vi "nxt main.vi"() -> ()   [LabVIEW 2012, in "Tugboat.lvrbt"]
uses:
  Tugboat.lvrbt
  tugProperties_t.ctl
  sensorData_t.ctl
  irData_t.ctl
  motorData_t.ctl
  motorCommands_t.ctl
  <vilib>/NXT/Block Support/NXT_TimerIndex.ctl
  behaviorWeights_t.ctl
panel:
  in  "_sendToPC":string
  in  "_fromPC":u8[](array[numeric])=[0, 0, 0, 0, 0, 0, 0, 0, 0, 0, 0]
  out "Sense/Act":bool=TRUE
  in  "_motorCommands":T1={"_rudderCommand"=7, "_propCommand"=7, "_irServoCommand"=7}
  in  "_motorData":T2={"_rudderCommand"=1450, "_propCommand"=1500, "_irServoCommand"=1550}
  in  "_sensorData":T3={"_irData"={"_irDistance"=0, "_irHeading"=0, "_irTimestamp"=0}, "_batteryVoltage"=0, "_NXTButtonStates"=[FALSE, FALSE, FALSE]}
  in  "Tugboat Properties":T5={"_name"="Enterprise", "_pitch"=440, "_rudderCenter"=1450, "_propCenter"=1500, "_irServoCenter"=1550, "_rudderMin"=930, "_rudderMax"=2000, "_propMin"=1000, "_propMax"=2000, "_irServoMin"=800, "_irServoMax"=2200}
  in  "SOFT E-STOP":bool
  in  "HARD E-STOP":bool
  # "L\nE\nF\nT"
  # "C\nE\nN\nT\nE\nR"
  # "R\nI\nG\nH\nT"
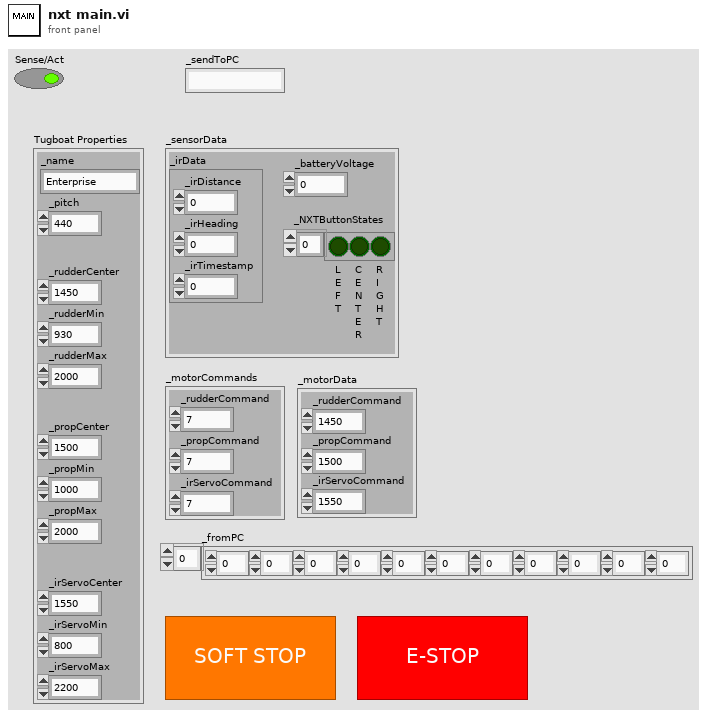
[diagram p1: front panel]
types:
  T1 = typedef "motorCommands_t.ctl" = cluster{"_rudderCommand":i8, "_propCommand":i8, "_irServoCommand":i8}
  T2 = typedef "motorData_t.ctl" = cluster{"_rudderCommand":u16, "_propCommand":u16, "_irServoCommand":u16}
  T3 = typedef "sensorData_t.ctl" = cluster{"_irData":T4, "_batteryVoltage":i32, "_NXTButtonStates":bool[]}
  T4 = typedef "irData_t.ctl" = cluster{"_irDistance":i32, "_irHeading":i32, "_irTimestamp":u32}
  T5 = typedef "tugProperties_t.ctl" = cluster{"_name":string, "_pitch":i32, "_rudderCenter":u16, "_propCenter":u16, "_irServoCenter":u16, "_rudderMin":u16, "_rudderMax":u16, "_propMin":u16, "_propMax":u16, "_irServoMin":u16, "_irServoMax":u16}
  T6 = typedef "behaviorWeights_t.ctl" = i8[]
  T7 = typedef "NXT_TimerIndex.ctl" = u8
  T8 = typedef "LVHSConnector.ctl" = cluster{"Hardware":string, "Flattened String":string}
  T9 = typedef "behaviorOutput_t.ctl" = cluster{"Goodness":i8[], "Velocity":i8[], "Weight":i8}
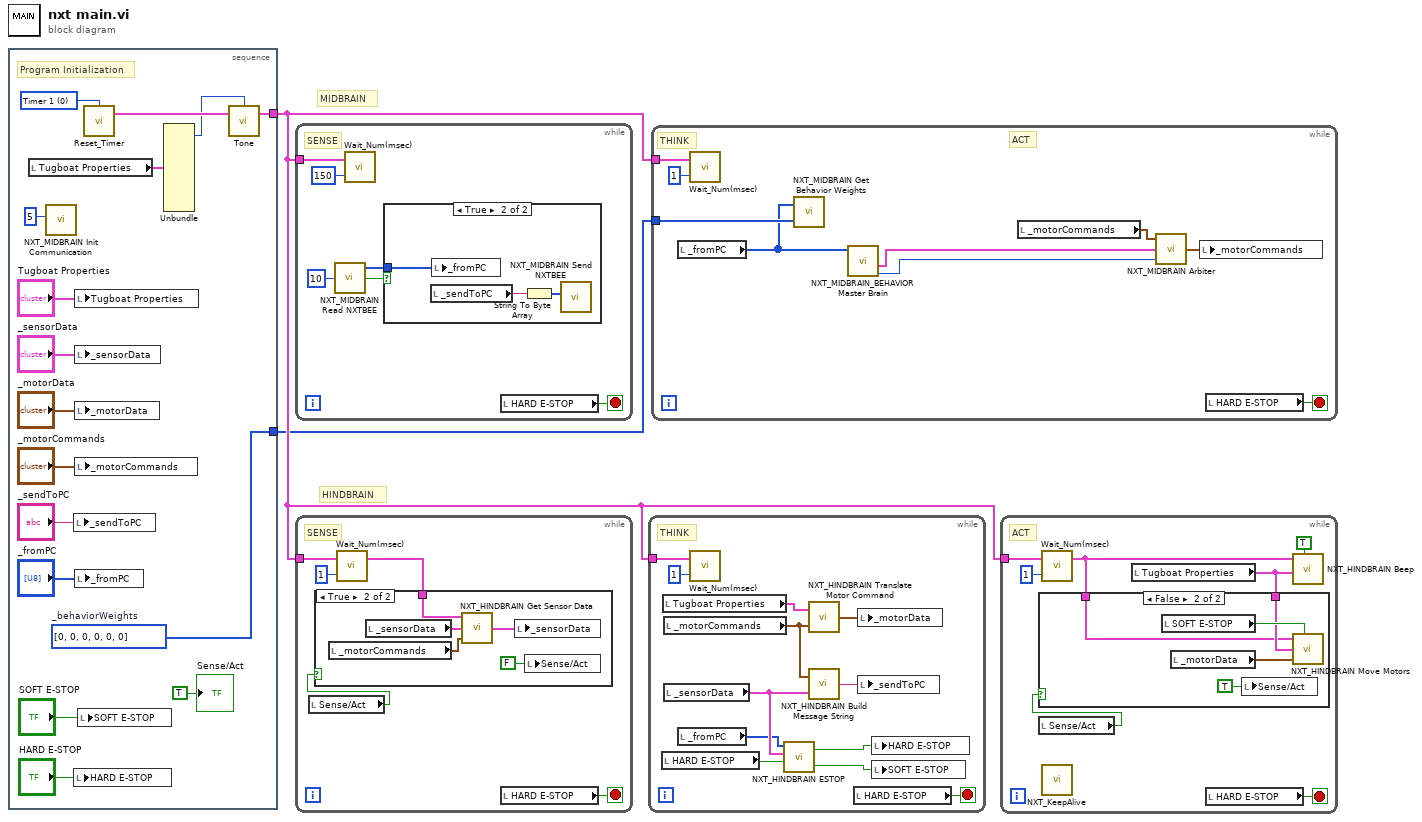
[diagram p0: block diagram]
diagram:
  # "HINDBRAIN"
  # "MIDBRAIN"
  n1 = stacked-sequence {
    tunnel: [w12] -> w2
    tunnel: [w6] -> w1
    frame #0 {
      w6 = T6 [0, 0, 0, 0, 0, 0]  # _behaviorWeights
      w14 = T7 0 items=["Timer 1", "Timer 2", "Timer 3"] ("Timer (Timer 1)")
      # "Program Initialization"
      n2 = local read "Tugboat Properties"() -> (w17:T5)
      n3 = call "NXT_MIDBRAIN Init Communication.vi"("Speed"=u8 5) -> ()  [unwired: 6 in, 1 out]
      n4 = local write "_sendToPC"("_sendToPC") -> ()
      n5 = local write "HARD E-STOP"("HARD E-STOP") -> ()
      n6 = local write "Tugboat Properties"("Tugboat Properties") -> ()
      n7 = local write "_sensorData"("_sensorData") -> ()
      n8 = local write "_motorData"("_motorData") -> ()
      n9 = local write "_motorCommands"("_motorCommands") -> ()
      n10 = local write "_fromPC"("_fromPC") -> ()
      n11 = local write "SOFT E-STOP"("SOFT E-STOP") -> ()
      n12 = call <vilib>:"Reset_Timer.vi"("Timer (Timer 1)"=w14) -> ("NXT"=w9:T8)  [unwired: 3 in]
      n13 = Unbundle(w17) -> ("_pitch"=w7:i32)  [unwired: 10 out]
      n14 = call <vilib>:"Tone.vi"("NXT"=w9, "Tone (440 Hz)"=w7) -> ("NXT"=w12:T8)  [unwired: 2 in]
      "Sense/Act" <- TRUE ("Sense/Act")
    }
  }
  n15 = while {
    tunnel: w2 -> [w23]
    stop <- w22 stop-if-true
    # "SENSE"
    n16 = call "NXT_MIDBRAIN Read NXTBEE.vi"("#bytes"=u8 10) -> ("Valid String?"=w19:bool, "Data Out"=w21:u8[])  [unwired: 2 in, 1 out]
    n17 = call <vilib>:"Wait_Num(msec).vi"("Time (100 msec)"=u32 150, "NXT"=w23) -> ()  [unwired: 2 in, 1 out]
    n18 = case shown="True" w19 {
      tunnel: w21 -> [_ w25]
      frame False {
      }
      frame True {
        n19 = local read "_sendToPC"() -> (w26:string)
        n20 = local write "_fromPC"(w25) -> ()
        n21 = String To Byte Array(string=w26) -> (unsigned byte array=w27:u8[])
        n22 = call "NXT_MIDBRAIN Send NXTBEE.vi"("Data"=w27) -> ()  [unwired: 8 in, 1 out]
      }
    }
    n23 = local read "HARD E-STOP"() -> (w22:bool)
  }
  n24 = while {
    tunnel: w2 -> [w29]
    stop <- w31 stop-if-true
    # "SENSE"
    n25 = local read "Sense/Act"() -> (w28:bool)
    n26 = call <vilib>:"Wait_Num(msec).vi"("Time (100 msec)"=u32 1, "NXT"=w29) -> ("NXT"=w30:T8)  [unwired: 2 in]
    n27 = case shown="True" w28 {
      tunnel: w30 -> [_ w37]
      frame False {
      }
      frame True {
        n28 = local read "_motorCommands"() -> (w35:T1)
        n29 = local read "_sensorData"() -> (w36:T3)
        n30 = call "NXT_HINDBRAIN Get Sensor Data.vi"("_motorCommands"=w35, "_sensorData"=w36, "NXT"=w37) -> ("_sensorData"=w34:T3)  [unwired: 2 in]
        n31 = local write "_sensorData"(w34) -> ()
        n32 = local write "Sense/Act"(FALSE ("Sense/Act")) -> ()
      }
    }
    n33 = local read "HARD E-STOP"() -> (w31:bool)
  }
  n34 = while {
    tunnel: w2 -> [w47]
    stop <- w48 stop-if-true
    # "THINK"
    n35 = local read "HARD E-STOP"() -> (w39:bool)
    n36 = local read "Tugboat Properties"() -> (w45:T5)
    n37 = local read "_motorCommands"() -> (w43:T1)
    n38 = local read "_sensorData"() -> (w42:T3)
    n39 = local read "_fromPC"() -> (w41:u8[])
    n40 = call <vilib>:"Wait_Num(msec).vi"("Time (100 msec)"=u32 1, "NXT"=w47) -> ()  [unwired: 2 in, 1 out]
    n41 = call "NXT_HINDBRAIN ESTOP.vi"("Hard E-Stop"=w39, "_sensorData"=w42, "_fromPC"=w41) -> ("Soft E-Stop"=w40:bool, "Hard E-Stop"=w46:bool)  [unwired: 1 in]
    n42 = call "NXT_HINDBRAIN Translate Motor Command.vi"("_motorCommands"=w43, "Tugboat Properties"=w45) -> ("_motorData"=w44:T2)
    n43 = call "NXT_HINDBRAIN Build Message String.vi"("_sensorData"=w42, "_motorCommands"=w43) -> ("Data Out"=w38:string)
    n44 = local read "HARD E-STOP"() -> (w48:bool)
    n45 = local write "_motorData"(w44) -> ()
    n46 = local write "_sendToPC"(w38) -> ()
    n47 = local write "HARD E-STOP"(w46) -> ()
    n48 = local write "SOFT E-STOP"(w40) -> ()
  }
  n49 = while {
    tunnel: w2 -> [w58]
    tunnel: w1 -> [w57]
    stop <- w53 stop-if-true
    # "ACT"
    # "THINK"
    n50 = local read "_fromPC"() -> (w52:u8[])
    n51 = call <vilib>:"Wait_Num(msec).vi"("Time (100 msec)"=u32 1, "NXT"=w58) -> ()  [unwired: 2 in, 1 out]
    n52 = call "NXT_MIDBRAIN Get Behavior Weights.vi"("_behaviorWeights"=w57, "_fromPC"=w52) -> ()  [unwired: 1 in, 1 out]
    n53 = call "NXT_MIDBRAIN_BEHAVIOR Master Brain.vi"("_behaviorWeights"=w52) -> ("_irTheta"=w50:i8, "_behaviorData"=w51:T9[])  [unwired: 5 in]
    n54 = local read "_motorCommands"() -> (w55:T1)
    n55 = call "NXT_MIDBRAIN Arbiter.vi"("_irServoCommand"=w50, "Behavior Data"=w51, "_motorCommands"=w55) -> ("_motorCommands"=w54:T1)
    n56 = local write "_motorCommands"(w54) -> ()
    n57 = local read "HARD E-STOP"() -> (w53:bool)
  }
  n58 = while {
    tunnel: w2 -> [w62]
    stop <- w63 stop-if-true
    # "ACT"
    n59 = local read "Sense/Act"() -> (w59:bool)
    n60 = call <vilib>:"Wait_Num(msec).vi"("Time (100 msec)"=u32 1, "NXT"=w62) -> ("NXT"=w60:T8)  [unwired: 2 in]
    n61 = call <vilib>:"NXT_KeepAlive.vi"() -> ()  [unwired: 10 in, 2 out]
    n62 = local read "Tugboat Properties"() -> (w61:T5)
    n63 = case shown="False" w59 {
      tunnel: w61 -> [_ w69]
      tunnel: w60 -> [_ w67]
      frame True {
      }
      frame False {
        n64 = local read "SOFT E-STOP"() -> (w70:bool)
        n65 = local read "_motorData"() -> (w68:T2)
        n66 = local write "Sense/Act"(TRUE ("Sense/Act")) -> ()
        n67 = call "NXT_HINDBRAIN Move Motors.vi"("NXT"=w67, "Motor Disable"=w70, "Tugboat Properties"=w69, "_motorData"=w68) -> ()  [unwired: 2 in]
      }
    }
    n68 = local read "HARD E-STOP"() -> (w63:bool)
    n69 = call "NXT_HINDBRAIN Beep.vi"("NXT"=w60, "Beep Enable"=TRUE, "Tugboat Properties"=w61) -> ()  [unwired: 3 in]
  }
